vi "GT Get Ext Io Bit.vi"(7 "pValue":u16, 8 "error in (no error)":errorcluster caption="错误输入（无错误）", 9 "index":i16, 10 "mdl":i16, 11 "cardNum":i16) -> (0 "error out":errorcluster caption="错误输出", 3 "function return":i16, 5 "pValue out":u16)   [LabVIEW 2020, in "gts.lvlib"]
doc: "GT_API GT_GetExtIoBit(short cardNum,short mdl,short index,unsigned short *pValue);"
uses:
  gts.lvlib
  dll/32bit/multi_card/gts.dll
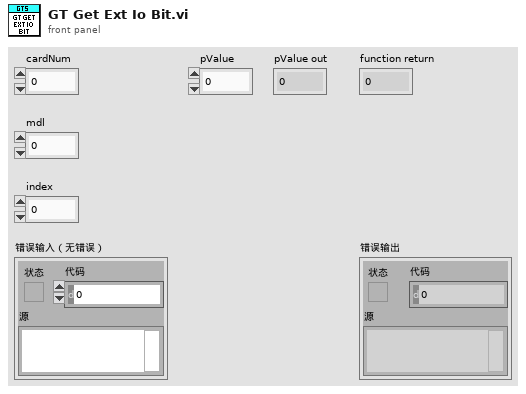
[diagram p1: front panel]
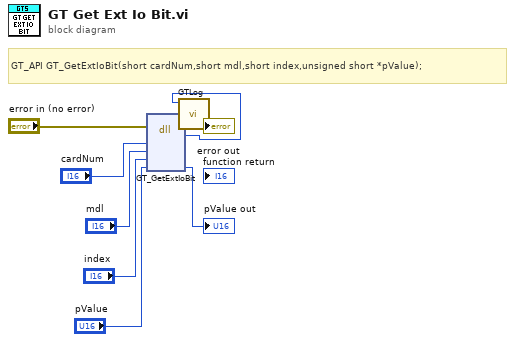
[diagram p0: block diagram]
diagram:
  # "GT_API GT_GetExtIoBit(short cardNum,short mdl,short index,unsigned short *pValue);"
  n1 = dll-call lib="C:/1228/dll/32bit/multi_card/gts.dll" fn="GT_GetExtIoBit"(error in="error in (no error)", "cardNum"="cardNum", "mdl"="mdl", "index"="index", "pValue"="pValue") -> (error out=w3:errorcluster, w1:i16, "pValue"=→"pValue out":u16)  [unwired: 5 in, 1 out]
  n2 = call "GTLog.vi"("error in (no error)"=w3, "Numeric"=w1) -> ("error out"=→"error out":errorcluster)  [unwired: 9 in]
